vi "TDSM2TDMLogPoly.vi"   [LabVIEW 2020]
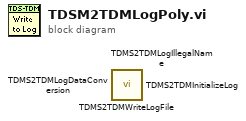
[diagram p0: block diagram]
diagram:
  n1 = call <vilib>:"TDMS2TDMWriteLogFile.vi"() -> ()  [unwired: 11 in, 1 out]
  n2 = call <vilib>:"TDMS2TDMLogIllegalName.vi"() -> ()  [unwired: 11 in, 1 out]
  n3 = call <vilib>:"TDMS2TDMLogDataConversion.vi"() -> ()  [unwired: 11 in, 1 out]
  n4 = call <vilib>:"TDMS2TDMInitializeLog.vi"() -> ()  [unwired: 9 in, 3 out]
